vi "zad1.vi"() -> ()   [LabVIEW 2018]
panel:
  out "Name":string
  in  "WebBrowser":refnum<k7>(container)
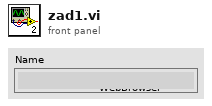
[diagram p1: front panel]
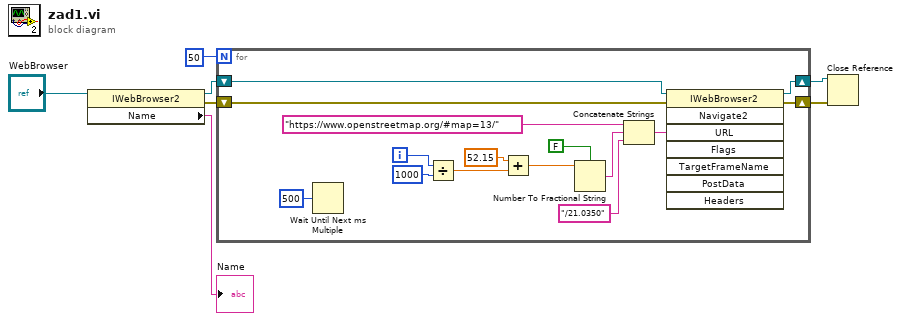
[diagram p0: block diagram]
diagram:
  n1 = property class="IWebBrowser2"(reference="WebBrowser") -> (reference out=w4:refnum<k7>, error out=w3:errorcluster, "Name"=→"Name":string)  [unwired: 1 in]
  n2 = for {
    N: 50 -> [_]
    shift-right: [w22] -> w7
    shift-left: w4 -> [w20]
    shift-right: [w21] -> w6
    shift-left: w3 -> [w19]
    i -> [w17]
    n3 = Wait Until Next ms Multiple(millisecond multiple=u32 500) -> ()  [unwired: 1 out]
    n4 = Divide(x=w17, y=1000) -> (x/y=w15:dbl)
    n5 = Add(x=52.15, y=w15) -> (x+y=w12:dbl)
    n6 = Number To Fractional String(use system decimal point (T)=FALSE, number=w12) -> (F-format string=w10:string)  [unwired: 2 in]
    n7 = Concatenate Strings("https://www.openstreetmap.org/#map=13/", w10, "/21.0350") -> (w9:string)
    n8 = invoke class="IWebBrowser2" method="Navigate2"(reference=w20, error in=w19, "URL"=w9) -> (reference out=w22:refnum<k7>, error out=w21:errorcluster)  [unwired: 5 in, 6 out]
  }
  n9 = Close Reference(reference=w7, error in (no error)=w6) -> ()  [unwired: 1 out]
